vi "Point Slope Calibration.vi"(11 "Error In":errorcluster) -> (4 "Pressure Slope":dbl, 6 "Pressure Intercept":dbl, 8 "Flow Array":dbl[](array[numeric]) format="%_6g", 15 "Error Out":errorcluster)   [LabVIEW 2013]
uses:
  <vilib>/Analysis/baseanly.llb/Mean (DBL).vi
  <vilib>/gmath/NI_Gmath.lvlib
  <vilib>/Analysis/NI_AALBase.lvlib
panel:
  out "Flow Calibration":cluster{"Y":dbl[], "Y":dbl[]}[](graph)
  in  "Pressure Reference":dbl min=0.0 max=20.0 step=4.0
  out "Pressure Voltage":dbl
  out "Flow Voltage":dbl
  in  "Flow Reference":dbl min=0.0 max=30.0 step=6.0
  out "Flow Intercept":dbl
  out "Flow Slope":dbl
  in  "Stop Button HS":bool
  in  "Add Button HS":bool
  out "Pressure Curve":cluster{"Y":dbl[], "Y":dbl[]}[](graph)
  out "Flow Curve":cluster{"Y":dbl[], "Y":dbl[]}[](graph)
  # "1. Connect the compressed air to the end of the pressure regulator.\n2. Connect the \"Before\" tube to the P+ port on the Flow side of the Amplifier.\n3. Connect the \"After\" tube to the P- port on.\n4. Connect the pressure calibrator unit to the P+ port on the Pressure side of the Amplifier.\n6. Record voltages and their corresponding pressures by clicking \"Add Value\"\n7. The slope and intercept will be saved for collection."
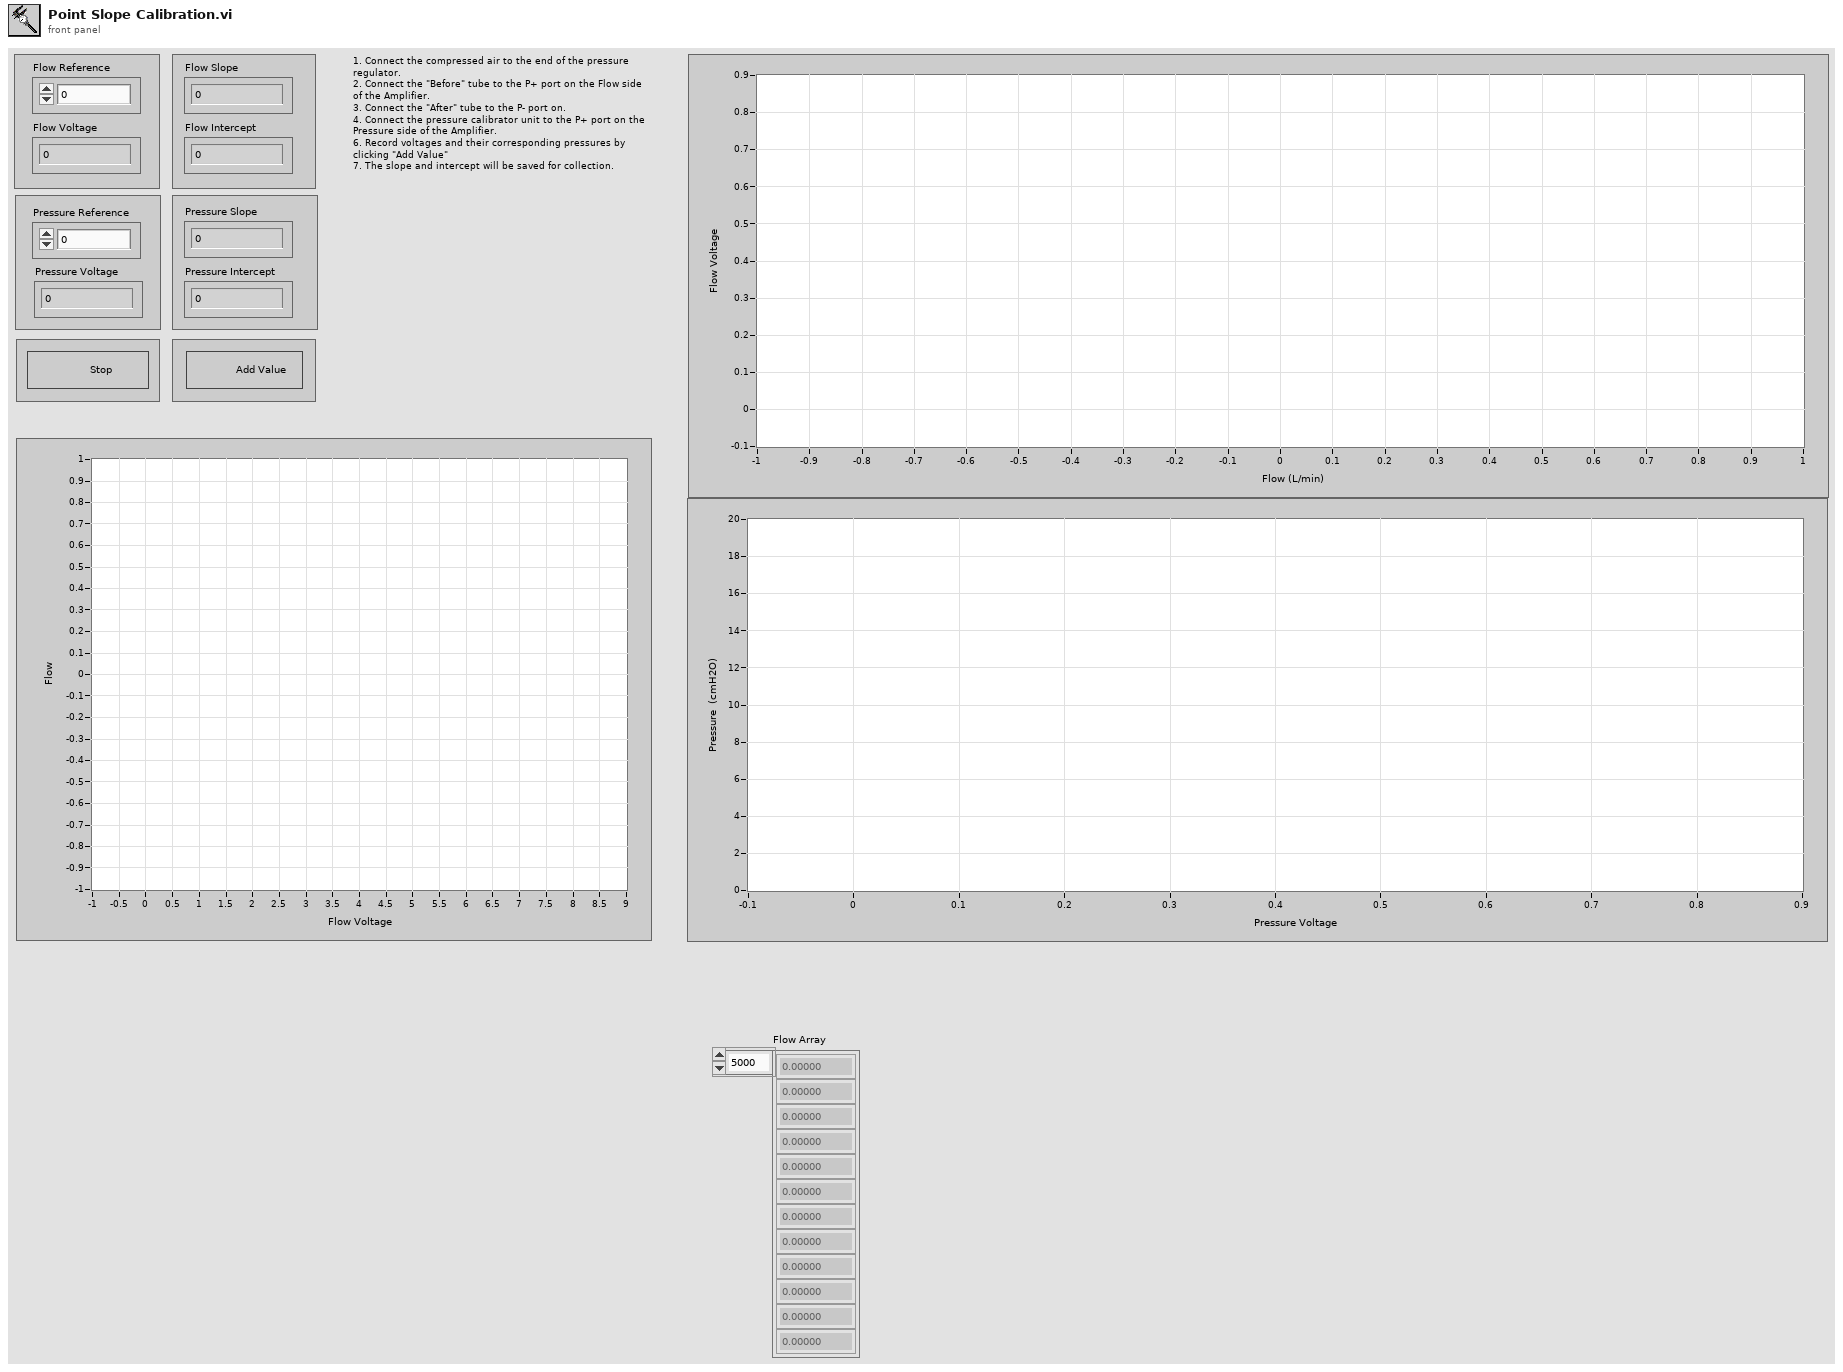
[diagram p1: front panel]
types:
  T1 = enum16{"open", "replace", "create", "open or create", "replace or create", "replace or create with confirmation"}
  T2 = enum8{"Enabled", "Disabled", "Disabled and Grayed Out"}
  T3 = cluster{"Volt (Flow)":dbl[], "Ref (Flow)":dbl[]}[]
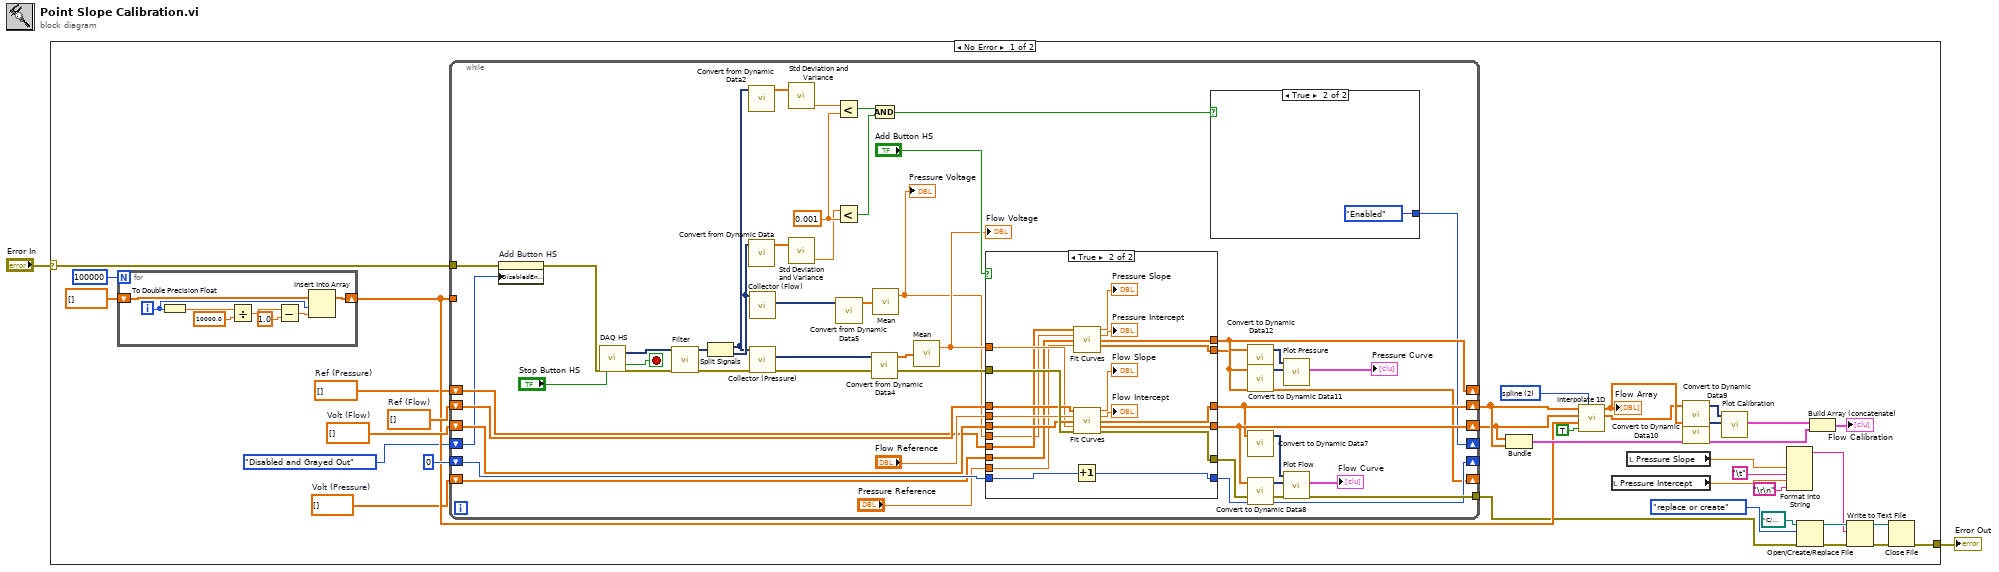
[diagram p0: block diagram]
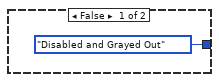
[diagram p2: hidden frame]
diagram:
  n1 = case shown="No Error" "Error In" {
    selector: "Error In" -> [w36 w121]
    tunnel: [w14 w121] -> w1
    frame No Error {
      w19 = dbl[] []  # Ref (Pressure)
      w20 = dbl[] []  # Volt (Pressure)
      w31 = 2 items=["nearest", "linear", "spline", "cubic Hermite", "Lagrange"] ("method")
      w34 = dbl[] []  # Ref (Flow)
      w35 = dbl[] []  # Volt (Flow)
      n2 = for {
        N: 100000 ("dimension size") -> [_]
        shift-right: [w43] -> w25
        shift-left: dbl[] [] -> [w44]
        i -> [w40]
        n3 = To Double Precision Float(number=w40) -> (double precision float=w41:dbl)
        n4 = Divide(x=w41, y=10000.0) -> (x/y=w39:dbl)
        n5 = Subtract(x=w39, y=1.0) -> (x-y=w37:dbl)
        n6 = Insert Into Array(array=w44, index=w40, new element=w37) -> (w43:dbl[])
      }
      n7 = while {
        tunnel: w36 -> [w60]
        shift-right: [w73] -> w17
        shift-left: w35 -> [w75]
        shift-right: [w72] -> w18
        shift-left: w34 -> [w77]
        tunnel: [w80] -> w15
        shift-right: [w78] -> _
        shift-left: 0 -> [w79]
        tunnel: w25 -> [_]
        shift-right: [w65] -> _
        shift-left: w20 -> [w67]
        shift-right: [w66] -> _
        shift-left: w19 -> [w68]
        shift-right: [w52] -> _
        shift-left: T2."Disabled and Grayed Out" ("Disabled") -> [w58]
        stop <- w87 stop-if-true
        w51 = 0.001
        n8 = property on="Add Button HS" class="Bool"(error in=w60, "DisabledEnum"=w58) -> (error out=w59:errorcluster)  [unwired: 1 in, 1 out]
        n9 = call "DAQ HS"("error in"=w59, "stop (F)"="Stop Button HS") -> ("data"=w91:dynamicdata, "stopped"=w87:bool, "error out"=w92:errorcluster)  [unwired: 14 in, 1 out]
        n10 = call "Filter"("error in (no error)"=w92, "Signal"=w91) -> ("error out"=w88:errorcluster, "Filtered Signal"=w70:dynamicdata)  [unwired: 8 in]
        n11 = Split Signals(w70) -> (w45:dynamicdata, w50:dynamicdata)  [unwired: 2 in]
        n12 = call "Convert from Dynamic Data2"("Dynamic Data Type"=w45) -> ("Array"=w49:dbl[])  [unwired: 3 in]
        n13 = call "Convert from Dynamic Data"("Dynamic Data Type"=w50) -> ("Array"=w48:dbl[])  [unwired: 3 in]
        n14 = call "Collector (Flow)"("Signals"=w50) -> ("Collected Signals"=w69:dynamicdata)  [unwired: 9 in, 1 out]
        n15 = call "Collector (Pressure)"("error in (no error)"=w88, "Signals"=w45) -> ("error out"=w84:errorcluster, "Collected Signals"=w86:dynamicdata)  [unwired: 8 in]
        n16 = call <vilib>:"Std Deviation and Variance.vi"("X"=w49) -> ("variance"=w46:dbl)  [unwired: 1 in, 2 out]
        n17 = call <vilib>:"Std Deviation and Variance.vi"("X"=w48) -> ("variance"=w47:dbl)  [unwired: 1 in, 2 out]
        n18 = Less?(x=w46, y=w51) -> (x < y?=w55:bool)
        n19 = Less?(x=w47, y=w51) -> (x < y?=w54:bool)
        n20 = call "Convert from Dynamic Data5"("Dynamic Data Type"=w69) -> ("Array"=w57:dbl[])  [unwired: 3 in]
        n21 = And(x=w55, y=w54) -> (x .and. y?=w53:bool)
        n22 = call "Convert from Dynamic Data4"("Dynamic Data Type"=w86) -> ("Array"=w85:dbl[])  [unwired: 3 in]
        n23 = call-poly <vilib>:"Mean.vi"("X"=w57) -> ("mean"=w56:dbl)  [unwired: 1 out]
        "Pressure Voltage" <- w56
        n24 = call-poly <vilib>:"Mean.vi"("X"=w85) -> ("mean"=w74:dbl)  [unwired: 1 out]
        "Flow Voltage" <- w74
        n25 = case shown="True" "Add Button HS" {
          tunnel: w84 -> [w100 w120]
          tunnel: [w100 w119] -> w83
          tunnel: w79 -> [w99 w118]
          tunnel: [w99 w117] -> w78
          tunnel: w77 -> [w98 w116]
          tunnel: "Flow Reference" -> [_ w115]
          tunnel: w75 -> [w97 w114]
          tunnel: w74 -> [_ w113]
          tunnel: [w98 w112] -> w72
          tunnel: [w97 w111] -> w73
          tunnel: "Pressure Reference" -> [_ w105]
          tunnel: w67 -> [w95 w104]
          tunnel: w68 -> [w96 w106]
          tunnel: w56 -> [_ w103]
          tunnel: [w96 w102] -> w66
          tunnel: [w95 w101] -> w65
          frame False {
          }
          frame True {
            n26 = Increment(x=w118) -> (x+1=w117:i32)
            n27 = call "Fit Curves.vi"("Reference (Array)"=w106, "Reference (Value)"=w103, "Voltage (Array)"=w104, "Voltage (Value)"=w105) -> ("Slope"=→"Pressure Slope":dbl, "Intercept"=→"Pressure Intercept":dbl, "Reference Out"=w102:dbl[], "Voltage Out"=w101:dbl[])  [unwired: 7 in, 1 out]
            n28 = call "Fit Curves.vi"("Reference (Array)"=w116, "Reference (Value)"=w115, "Voltage (Array)"=w114, "Voltage (Value)"=w113, "Error In"=w120) -> ("Slope"=→"Flow Slope":dbl, "Intercept"=→"Flow Intercept":dbl, "Reference Out"=w112:dbl[], "Voltage Out"=w111:dbl[], "Error Out"=w119:errorcluster)  [unwired: 6 in]
          }
        }
        n29 = case shown="True" w53 {
          tunnel: [T2."Disabled and Grayed Out" ("Disabled") T2."Enabled" ("Disabled")] -> w52
          frame False {
          }
          frame True {
          }
        }
        n30 = call "Convert to Dynamic Data12"("Array"=w66) -> ("Dynamic Data Type"=w64:dynamicdata)  [unwired: 3 in]
        n31 = call "Convert to Dynamic Data11"("Array"=w65) -> ("Dynamic Data Type"=w63:dynamicdata)  [unwired: 3 in]
        n32 = call "Convert to Dynamic Data7"("Array"=w72) -> ("Dynamic Data Type"=w81:dynamicdata)  [unwired: 3 in]
        n33 = call "Convert to Dynamic Data8"("Array"=w73) -> ("Dynamic Data Type"=w82:dynamicdata)  [unwired: 3 in]
        n34 = call "Plot Pressure"("Y Input"=w63, "X Input"=w64) -> ("XY Graph"=→"Pressure Curve":cluster{"Y":dbl[], "Y":dbl[]}[])  [unwired: 8 in, 1 out]
        n35 = call "Plot Flow"("error in (no error)"=w83, "Y Input"=w82, "X Input"=w81) -> ("error out"=w80:errorcluster, "XY Graph"=→"Flow Curve":cluster{"Y":dbl[], "Y":dbl[]}[])  [unwired: 7 in]
      }
      n36 = Bundle("Volt (Flow)"=w17, "Ref (Flow)"=w18) -> (w27:cluster{"Volt (Flow)":dbl[], "Ref (Flow)":dbl[]})  [unwired: 1 in]
      n37 = call <vilib>:"Interpolate 1D.vi"("method"=w31, "X is monotonic"=TRUE, "xi"=w25, "X"=w17, "Y"=w18) -> ("xi used"=w22:dbl[], "yi"=w23:dbl[])  [unwired: 4 in, 1 out]
      "Flow Array" <- w23
      n38 = local read "Pressure Intercept"() -> (w3:dbl)
      n39 = local read "Pressure Slope"() -> (w4:dbl)
      n40 = call "Convert to Dynamic Data9"("Array"=w22) -> ("Dynamic Data Type"=w30:dynamicdata)  [unwired: 3 in]
      n41 = call "Convert to Dynamic Data10"("Array"=w23) -> ("Dynamic Data Type"=w29:dynamicdata)  [unwired: 3 in]
      n42 = call "Plot Calibration"("Y Input"=w29, "X Input"=w30) -> ("XY Graph"=w28:cluster{"Y":dbl[], "Y":dbl[]}[])  [unwired: 8 in, 1 out]
      n43 = Format Into String(w4, "\t", w3, "\r\n") -> (resulting string=w7:string)  [unwired: 3 in, 1 out]
      n44 = Open/Create/Replace File(file path (use dialog)=path "C:/Users/scholp/Desktop/Stand-Alone Calibration/Calibration Values.txt", error in=w15, operation (0:open)=T1."replace or create") -> (refnum out=w11:refnum<file>, error out=w12:errorcluster)  [unwired: 3 in, 1 out]
      n45 = Build Array (concatenate)(w28, w27) -> (→"Flow Calibration":T3)
      n46 = Write to Text File(file (use dialog)=w11, text=w7, error in=w12) -> (refnum out=w10:refnum<file>, error out=w13:errorcluster)  [unwired: 1 in, 1 out]
      n47 = Close File(refnum=w10, error in=w13) -> (error out=w14:errorcluster)  [unwired: 1 out]
    }
    frame Error {
    }
  }
  "Error Out" <- w1
